vi "METIS control v0.1.vi"() -> ()   [LabVIEW 2018]
uses:
  <userlib>/caLab/Private/Put_String_PV.vi
  <userlib>/caLab/Private/Put_I16_PV.vi
  <userlib>/caLab/Private/Get_PV.vi
panel:
  out "Extractor current":dbl(graph)=1.03335
  out "Custom 1D 2 Counts":dbl(graph)=1.0
  in  "Boolean 6":bool
  in  "Boolean 5":bool
  in  "Boolean 4":bool
  in  "Boolean 3":bool
  in  "Boolean 2":bool
  in  "Boolean":bool
  out "Intensity Graph 6":dbl[][](graph)
  out "Intensity Graph 5":dbl[][](graph)
  out "Intensity Graph 4":dbl[][](graph)
  out "Intensity Graph 3":dbl[][](graph)
  out "Intensity Graph 2":dbl[][](graph)
  out "Countrate":dbl=111924.0 format="%#_5e"
  out "Metis Countrate":dbl(graph)=111924.0
  out "Intensity Graph":dbl[][](graph)
  in  "Reset":bool
  out "AccumTimeInCube_RBV":dbl=35.0
  in  "Stop Acquire":bool
  in  "Start Acquire":bool
  out "Acquire":string="Acquire"
  in  "stop":bool
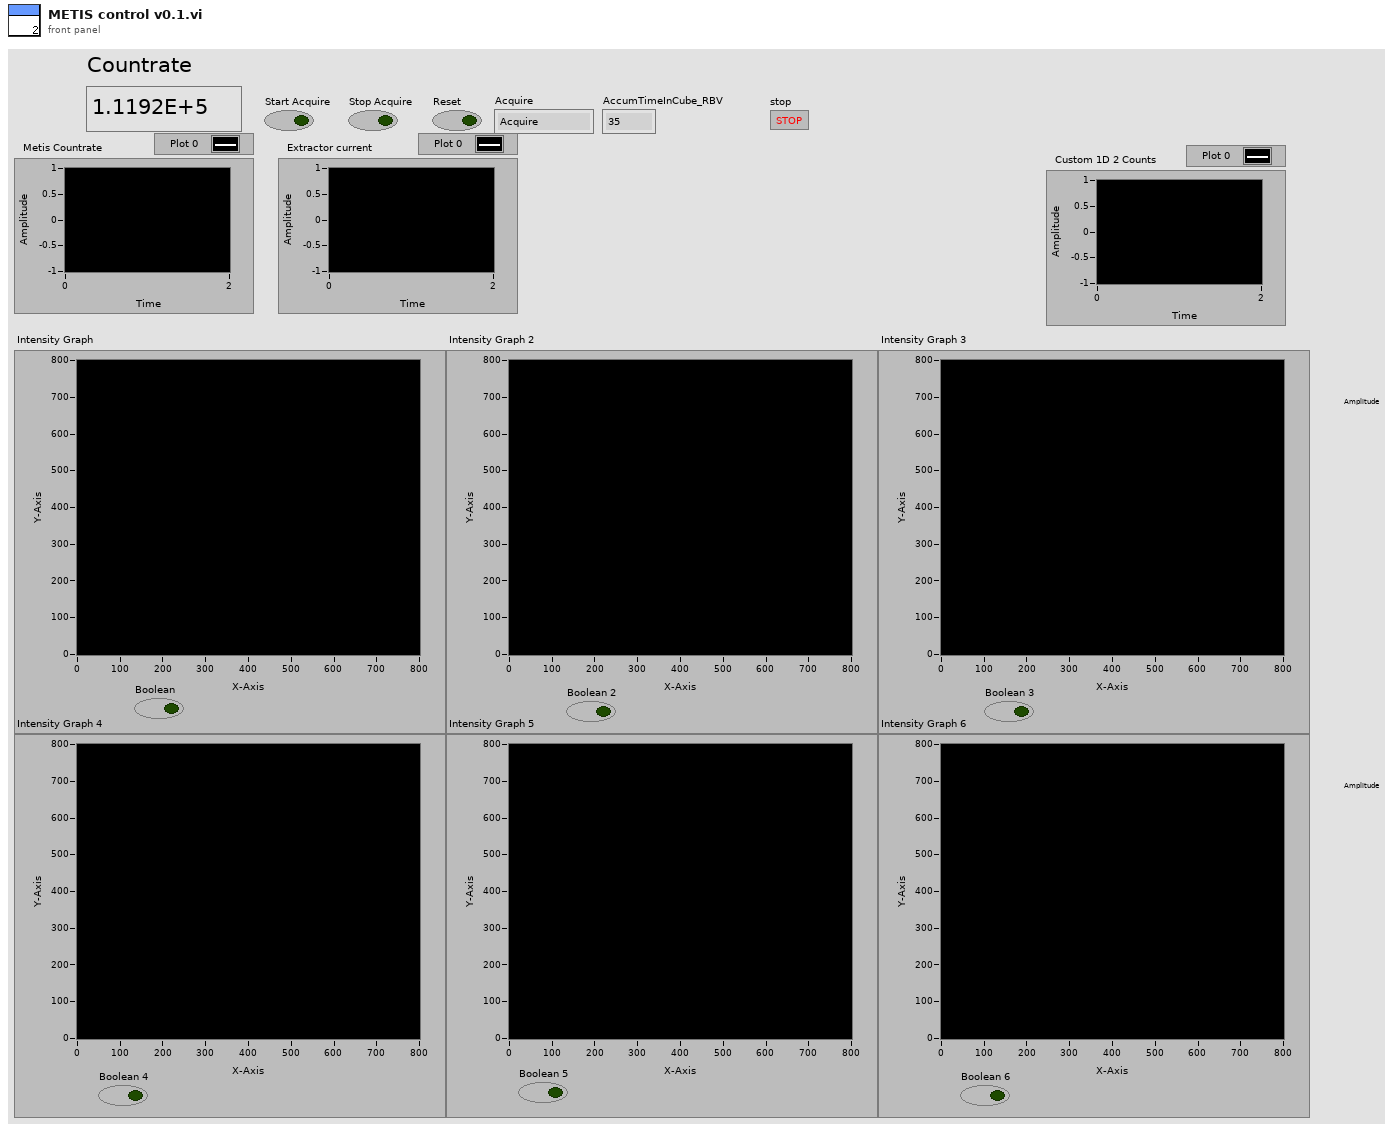
[diagram p1: front panel]
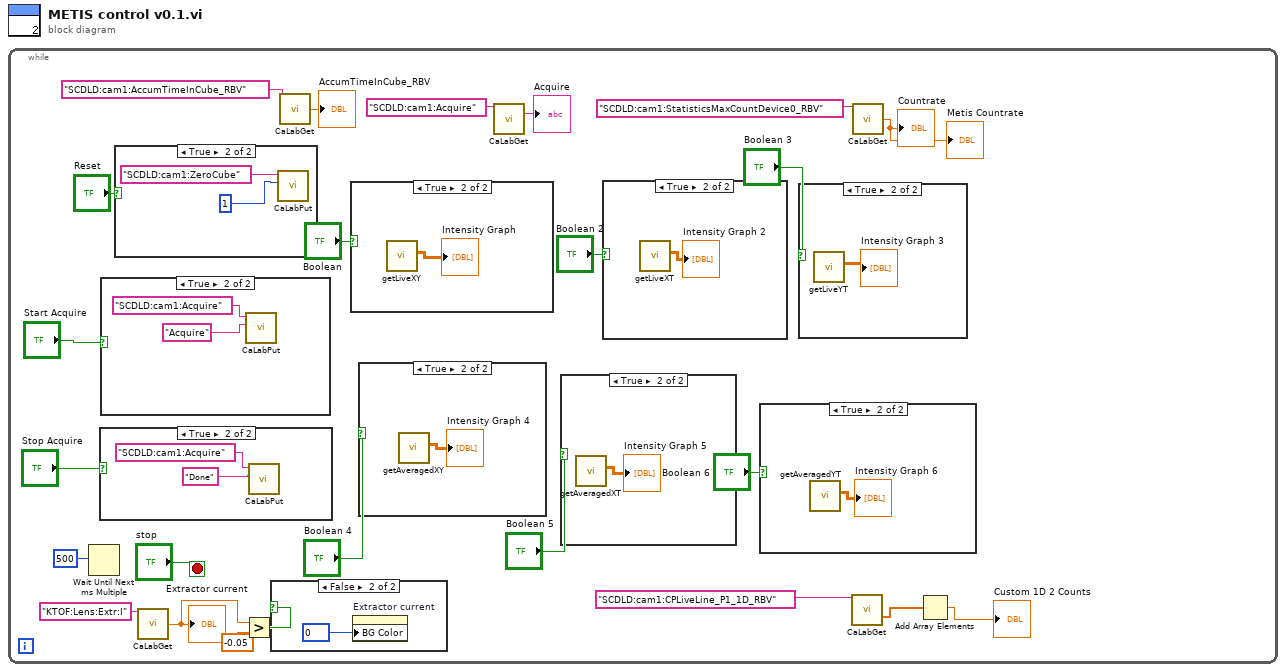
[diagram p0: block diagram]
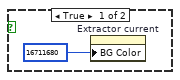
[diagram p2: hidden frame]
diagram:
  n1 = while {
    stop <- "stop" stop-if-true
    n2 = Wait Until Next ms Multiple(millisecond multiple=u32 500 ("milliseconds to wait")) -> ()  [unwired: 1 out]
    n3 = case shown="True" "Stop Acquire" {
      frame False {
      }
      frame True {
        n4 = call-poly <userlib>:"CaLabPut.vi"("Value"="Done" ("VAL"), "PV Name"="SCDLD:cam1:Acquire") -> ()  [unwired: 6 in, 4 out]
      }
    }
    n5 = case shown="True" "Start Acquire" {
      frame False {
      }
      frame True {
        n6 = call-poly <userlib>:"CaLabPut.vi"("Value"="Acquire" ("VAL"), "PV Name"="SCDLD:cam1:Acquire") -> ()  [unwired: 6 in, 4 out]
      }
    }
    n7 = case shown="True" "Reset" {
      frame False {
      }
      frame True {
        n8 = call-poly <userlib>:"CaLabPut.vi"("Value"=i16 1 ("ZeroCube"), "PV Name"="SCDLD:cam1:ZeroCube") -> ()  [unwired: 6 in, 4 out]
      }
    }
    n9 = call-poly <userlib>:"CaLabGet.vi"("PV Name"="KTOF:Lens:Extr:I") -> ("1rst Value (number)"=w3:dbl)  [unwired: 8 in, 6 out]
    "Extractor current" <- w3
    n10 = Greater?(x=w3, y=-0.05) -> (0:w1:bool)
    n11 = case shown="False" w1 {
      frame True {
        n12 = property on="Extractor current" class="WFChart (strict)"("BG Color"=u32 16711680 ("Plot Area:Colors:BG Color")) -> ()  [unwired: 2 in, 2 out]
      }
      frame False {
        n13 = property on="Extractor current" class="WFChart (strict)"("BG Color"=u32 0 ("Plot Area:Colors:BG Color")) -> ()  [unwired: 2 in, 2 out]
      }
    }
    n14 = call-poly <userlib>:"CaLabGet.vi"("PV Name"="SCDLD:cam1:AccumTimeInCube_RBV") -> ("1rst Value (number)"=→"AccumTimeInCube_RBV":dbl)  [unwired: 8 in, 6 out]
    n15 = case shown="True" "Boolean" {
      frame False {
      }
      frame True {
        n16 = call "getLiveXY.vi"() -> ("transposed array"=→"Intensity Graph":dbl[][])  [unwired: 3 out]
      }
    }
    n17 = case shown="True" "Boolean 4" {
      frame False {
      }
      frame True {
        n18 = call "getAveragedXY.vi"() -> ("transposed array"=→"Intensity Graph 4":dbl[][])  [unwired: 3 out]
      }
    }
    n19 = call-poly <userlib>:"CaLabGet.vi"("PV Name"="SCDLD:cam1:Acquire") -> ("1rst Value (string)"=→"Acquire":string)  [unwired: 8 in, 6 out]
    n20 = case shown="True" "Boolean 5" {
      frame False {
      }
      frame True {
        n21 = call "getAveragedXT.vi"() -> ("transposed array"=→"Intensity Graph 5":dbl[][])  [unwired: 3 out]
      }
    }
    n22 = case shown="True" "Boolean 2" {
      frame False {
      }
      frame True {
        n23 = call "getLiveXT.vi"() -> ("transposed array"=→"Intensity Graph 2":dbl[][])  [unwired: 3 out]
      }
    }
    n24 = case shown="True" "Boolean 6" {
      frame False {
      }
      frame True {
        n25 = call "getAveragedYT.vi"() -> ("transposed array"=→"Intensity Graph 6":dbl[][])  [unwired: 3 out]
      }
    }
    n26 = case shown="True" "Boolean 3" {
      frame False {
      }
      frame True {
        n27 = call "getLiveYT.vi"() -> ("transposed array"=→"Intensity Graph 3":dbl[][])  [unwired: 3 out]
      }
    }
    n28 = call-poly <userlib>:"CaLabGet.vi"("PV Name"="SCDLD:cam1:CPLiveLine_P1_1D_RBV") -> ("Value Array (number)"=w7:dbl[])  [unwired: 8 in, 6 out]
    n29 = call-poly <userlib>:"CaLabGet.vi"("PV Name"="SCDLD:cam1:StatisticsMaxCountDevice0_RBV") -> ("1rst Value (number)"=→"Metis Countrate" →"Countrate":dbl)  [unwired: 8 in, 6 out]
    n30 = Add Array Elements(numeric array=w7) -> (sum=→"Custom 1D 2 Counts":dbl)
  }
